vi "Example OpenCV Object Tracking 1.0.vi"() -> ()   [LabVIEW 2014]
uses:
  vi.lib/Q-WaveSystems/QwaveSys Raspberry Pi for LabVIEW Home-Education/QwaveSys Raspberry Pi Library.lvlib
panel:
  out "return type":i32
  out "found":u32[][](array[numeric])
  in  "webcamnum":i32
  in  "Color Upper":T1={"Lower H"=160, "Lower S"=100, "Lower V"=100, "Upper H"=180, "Upper S"=255, "Upper V"=255}
  in  "Color Lower":T1={"Lower H"=0, "Lower S"=100, "Lower V"=100, "Upper H"=25, "Upper S"=255, "Upper V"=255}
  out "Output":picture
  in  "Blank Button":bool
  out "2D Picture":picture
  # "R"
  # "Y"
  # "X"
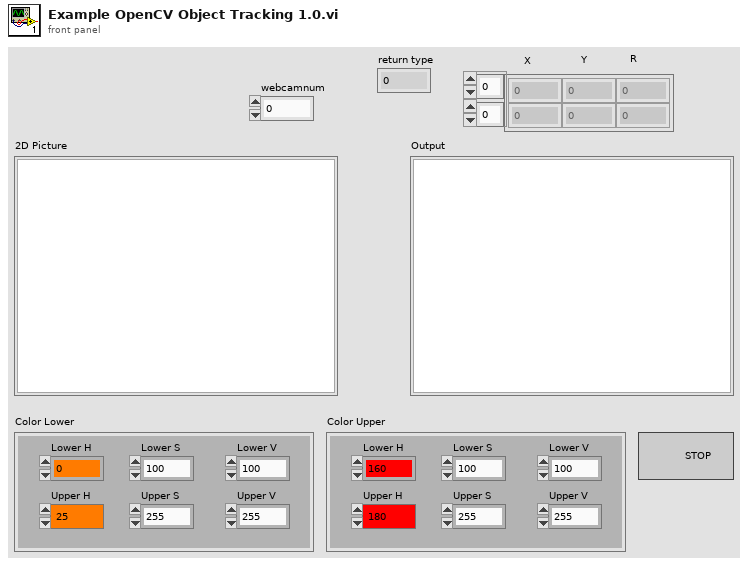
[diagram p1: front panel]
types:
  T1 = cluster{"Lower H":u8, "Lower S":u8, "Lower V":u8, "Upper H":u8, "Upper S":u8, "Upper V":u8}
  T2 = typedef "imagedata.ctl" = cluster{"image type":i32, "image depth":i32, "image":u8[], "mask":u8[], "colors":u32[], "Rectangle":cluster{"left":i16, "top":i16, "right":i16, "bottom":i16}}
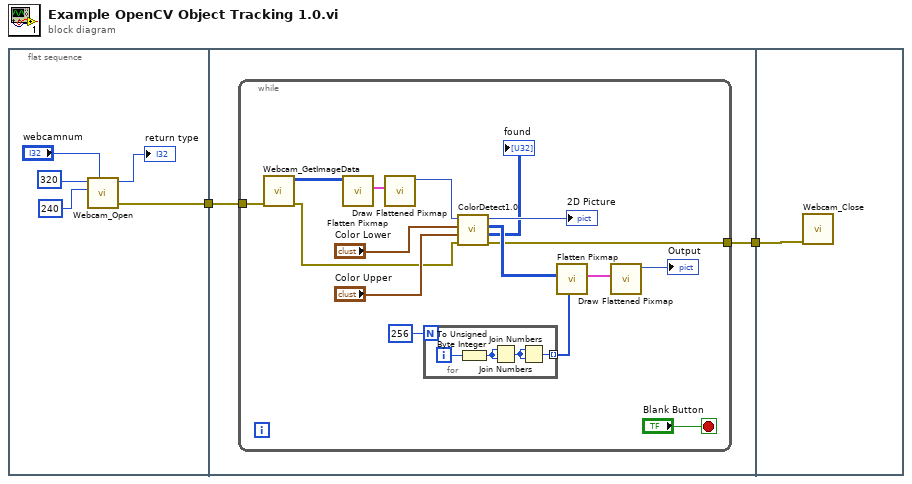
[diagram p0: block diagram]
diagram:
  n1 = flat-sequence {
    tunnel: [w4] -> w2
    tunnel: w2 -> [w9]
    tunnel: [w8] -> w1
    tunnel: w1 -> [w30]
    frame #0 {
      n2 = call "Webcam_Open.vi"("webcamnum"="webcamnum", "height"=u32 240, "width"=u32 320) -> ("error out"=w4:errorcluster, "return type"=→"return type":i32)  [unwired: 7 in]
    }
    frame #1 {
      n3 = while {
        tunnel: w9 -> [w12]
        tunnel: [w10] -> w8
        stop <- "Blank Button" stop-if-true
        n4 = call "Webcam_GetImageData.vi"("error in (no error)"=w12) -> ("error out"=w11:errorcluster, "image24bits"=w19:u32[][])  [unwired: 8 in, 1 out]
        n5 = call <vilib>:"Flatten Pixmap.vi"("24-bit pixmap"=w19) -> ("image data"=w25:T2)  [unwired: 10 in]
        n6 = call <vilib>:"Draw Flattened Pixmap.vi"("image data"=w25) -> ("new picture"=w18:picture)  [unwired: 8 in]
        n7 = for {
          N: 256 -> [_]
          tunnel: [w29] -> w20 mode=indexing
          i -> [w27]
          n8 = To Unsigned Byte Integer(number=w27) -> (unsigned 8bit integer=w26:u8)
          n9 = Join Numbers(hi=w26, lo=w26) -> ((hi.lo)=w28:u16)
          n10 = Join Numbers(hi=w28, lo=w28) -> ((hi.lo)=w29:u32)
        }
        n11 = call "ColorDetect1.0.vi"("error in (no error)"=w11, "Color Upper"="Color Upper", "Color Lower"="Color Lower", "new picture"=w18) -> ("error out"=w10:errorcluster, "found"=→"found":u32[][], "image"=w14:u8[][], "out picture"=→"2D Picture":picture)  [unwired: 4 in]
        n12 = call <vilib>:"Flatten Pixmap.vi"("colors"=w20, "8-bit pixmap"=w14) -> ("image data"=w23:T2)  [unwired: 9 in]
        n13 = call <vilib>:"Draw Flattened Pixmap.vi"("image data"=w23) -> ("new picture"=→"Output":picture)  [unwired: 8 in]
      }
    }
    frame #2 {
      n14 = call "Webcam_Close.vi"("error in (no error)"=w30) -> ()  [unwired: 10 in, 1 out]
    }
  }
